vi "MGCC_MdlMgmt_string_to_complex.vi"(1 "String Input":string) -> (0 "Complex Number":cdb)   [LabVIEW 2016]
doc: "Takes a string input in one of the following formats:\nx+iy, -x+iy, x-iy, -x-iy, x+jy, -x+jy, x-jy, -x-jy, where x and y are numbers.\n\nThe VI then splits the sting into three strings: the real part (including the middle operator), the i or j, and complex part. Next, the \"+\" or \"-\" case is selected by extracting the last element of the string containing the real part. The extraction is done by determining the length-1 of the string and making this value the offset for String Subset, which leaves just the operator as the substring for the case selector. Inside the cases, the string are converted to double precision numbers and combined into a complex number. The \"-\" case converts the complex part to a negaitve number by subtracting it from zero."
panel:
  in  "Use \"i\" or \"j\"?":string="i"
  # "Overview: The VI converts the string format with complex numbers to complex number format.\n\nRequirements: LabVIEW 2012 (or compatible).\n\nInstructions:\n1. Insert string input.\n2. Run the VI.\n3, Write down the result from Complex Number."
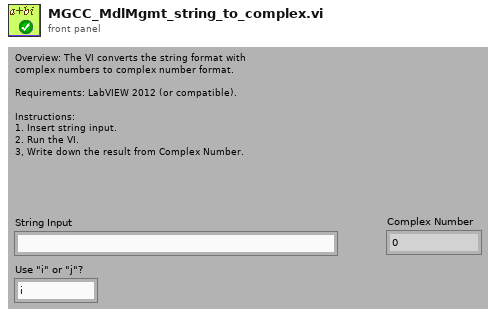
[diagram p1: front panel]
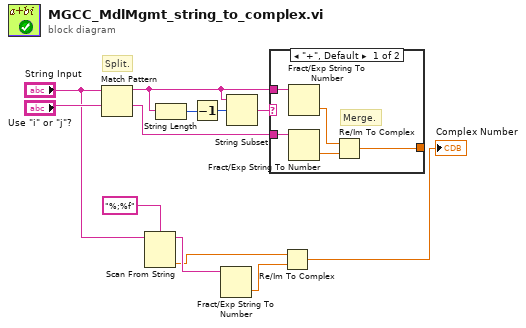
[diagram p0: block diagram]
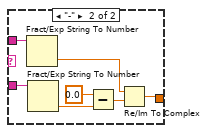
[diagram p2: hidden frame]
diagram:
  # "Split."
  n1 = Match Pattern(string="String Input", regular expression="Use \"i\" or \"j\"?") -> (before substring=w9:string, after substring=w12:string)  [unwired: 3 out]
  n2 = Scan From String(format string="%;%f", input string="String Input") -> (remaining string=w4:string, output 1=w3:dbl)  [unwired: 3 in, 2 out]
  n3 = String Length(string=w9) -> (length=w10:i32)
  n4 = Decrement(x=w10) -> (x-1=w8:i32)
  n5 = Fract/Exp String To Number(string=w4) -> (number=w2:dbl)  [unwired: 3 in, 1 out]
  n6 = String Subset(string=w9, offset (0)=w8) -> (substring=w11:string)  [unwired: 1 out]
  n7 = case shown="\"+\", Default" w11 {
    tunnel: w9 -> [w15 w24]
    tunnel: w12 -> [w14 w18]
    tunnel: [w13 w19] -> _
    frame "+", Default {
      # "Merge."
      n8 = Fract/Exp String To Number(string=w15) -> (number=w16:dbl)  [unwired: 4 out]
      n9 = Fract/Exp String To Number(string=w14) -> (number=w17:dbl)  [unwired: 4 out]
      n10 = Re/Im To Complex(1:w17, 2:w16) -> (0:w13:cdb)
    }
    frame "-" {
      n11 = Fract/Exp String To Number(string=w24) -> (number=w23:dbl)  [unwired: 4 out]
      n12 = Fract/Exp String To Number(string=w18) -> (number=w20:dbl)  [unwired: 4 out]
      n13 = Subtract(x=0.0, y=w20) -> (x-y=w22:dbl)
      n14 = Re/Im To Complex(1:w22, 2:w23) -> (0:w19:cdb)
    }
  }
  n15 = Re/Im To Complex(1:w2, 2:w3) -> (0:→"Complex Number":cdb)
